vi "EncoderForward.vi"(8 "EncoderDevRef 4":T2={"DevStatus"={"status"=FALSE, "code"=0, "source"=""}, "EncoderIndex"=enum."Invalid", "CounterIndex"=enum."Ctr 1", "DistancePerCount"=2.0, "Decoding Type"=enum."4x"}, 9 "RobotDriveDevRef":T6={"DevStatus"={"status"=FALSE, "code"=0, "source"=""}, "Motors[]"=[], "Square Inputs"=FALSE, "Max Output"=1.0, "Isochronous"=FALSE}, 10 "EncoderDevRef":T2={"DevStatus"={"status"=FALSE, "code"=0, "source"=""}, "EncoderIndex"=enum."Invalid", "CounterIndex"=enum."Ctr 1", "DistancePerCount"=2.0, "Decoding Type"=enum."4x"}, 11 "Target":dbl format="%#_13g") -> (0 "EncoderDevRef 3":T2={"DevStatus"={"status"=FALSE, "code"=0, "source"=""}, "EncoderIndex"=enum."Invalid", "CounterIndex"=enum."Ctr 1", "DistancePerCount"=2.0, "Decoding Type"=enum."4x"}, 1 "RobotDriveDevRef 2":T6={"DevStatus"={"status"=FALSE, "code"=0, "source"=""}, "Motors[]"=[], "Square Inputs"=FALSE, "Max Output"=1.0, "Isochronous"=FALSE}, 2 "EncoderDevRef 2":T2={"DevStatus"={"status"=FALSE, "code"=0, "source"=""}, "EncoderIndex"=enum."Invalid", "CounterIndex"=enum."Ctr 1", "DistancePerCount"=2.0, "Decoding Type"=enum."4x"})   [LabVIEW 2013]
uses:
  <vilib>/Rock Robotics/WPI/RobotDrive/WPI_RobotDriveDevRef.ctl
  <vilib>/Rock Robotics/WPI/MotorControl/WPI_MotorControlDeviceRef.ctl
  <vilib>/Rock Robotics/SystemInterfaces/Typedef/FPGA_TypedefDigitalModule.ctl
  <vilib>/Rock Robotics/SystemInterfaces/DIO/FPGA_DIOPWMChannel.ctl
  <vilib>/Rock Robotics/WPI/PWM/WPI_PWMDeadband.ctl
  <vilib>/Rock Robotics/WPI/CAN/Jaguar/SubVIs/WPI_CANJaguar_ControlMode.ctl
  <vilib>/Rock Robotics/WPI/PWM/WPI_PWMTransform_ConPane.ctl
  <vilib>/Rock Robotics/WPI/Encoder/WPI_EncoderDevRef.ctl
  <vilib>/Rock Robotics/SystemInterfaces/Encoder/FPGA_EncoderIdx.ctl
  <vilib>/Rock Robotics/SystemInterfaces/Counter/FPGA_CounterCtrSystemIndex.ctl
  <vilib>/Rock Robotics/WPI/Encoder/WPI_EncoderType.ctl
  <vilib>/addons/control/pid/pid.llb/PID (DBL).vi
  <vilib>/addons/control/pid/NI_PID_pid.lvlib
panel:
  out "dt out (s)":dbl format="%.3f"
  out "Right Distance":dbl(graph)
  out "Right Motor Power":dbl(graph)
  out "Left Motor Power":dbl(graph)
  out "Left Distance":dbl(graph)
  in  "PID gains 3":T1={"proportional gain (Kc)"=0.15, "integral time (Ti, min)"=0.0, "derivative time (Td, min)"=0.0}
  in  "output range 3":cluster{"output high":dbl, "output low":dbl}={"output high"=1.0, "output low"=-1.0}
  in  "output range 2":cluster{"output high":dbl, "output low":dbl}={"output high"=1.0, "output low"=-1.0}
  in  "PID gains 2":T1={"proportional gain (Kc)"=0.15, "integral time (Ti, min)"=0.0, "derivative time (Td, min)"=0.0}
  # "Stop?"
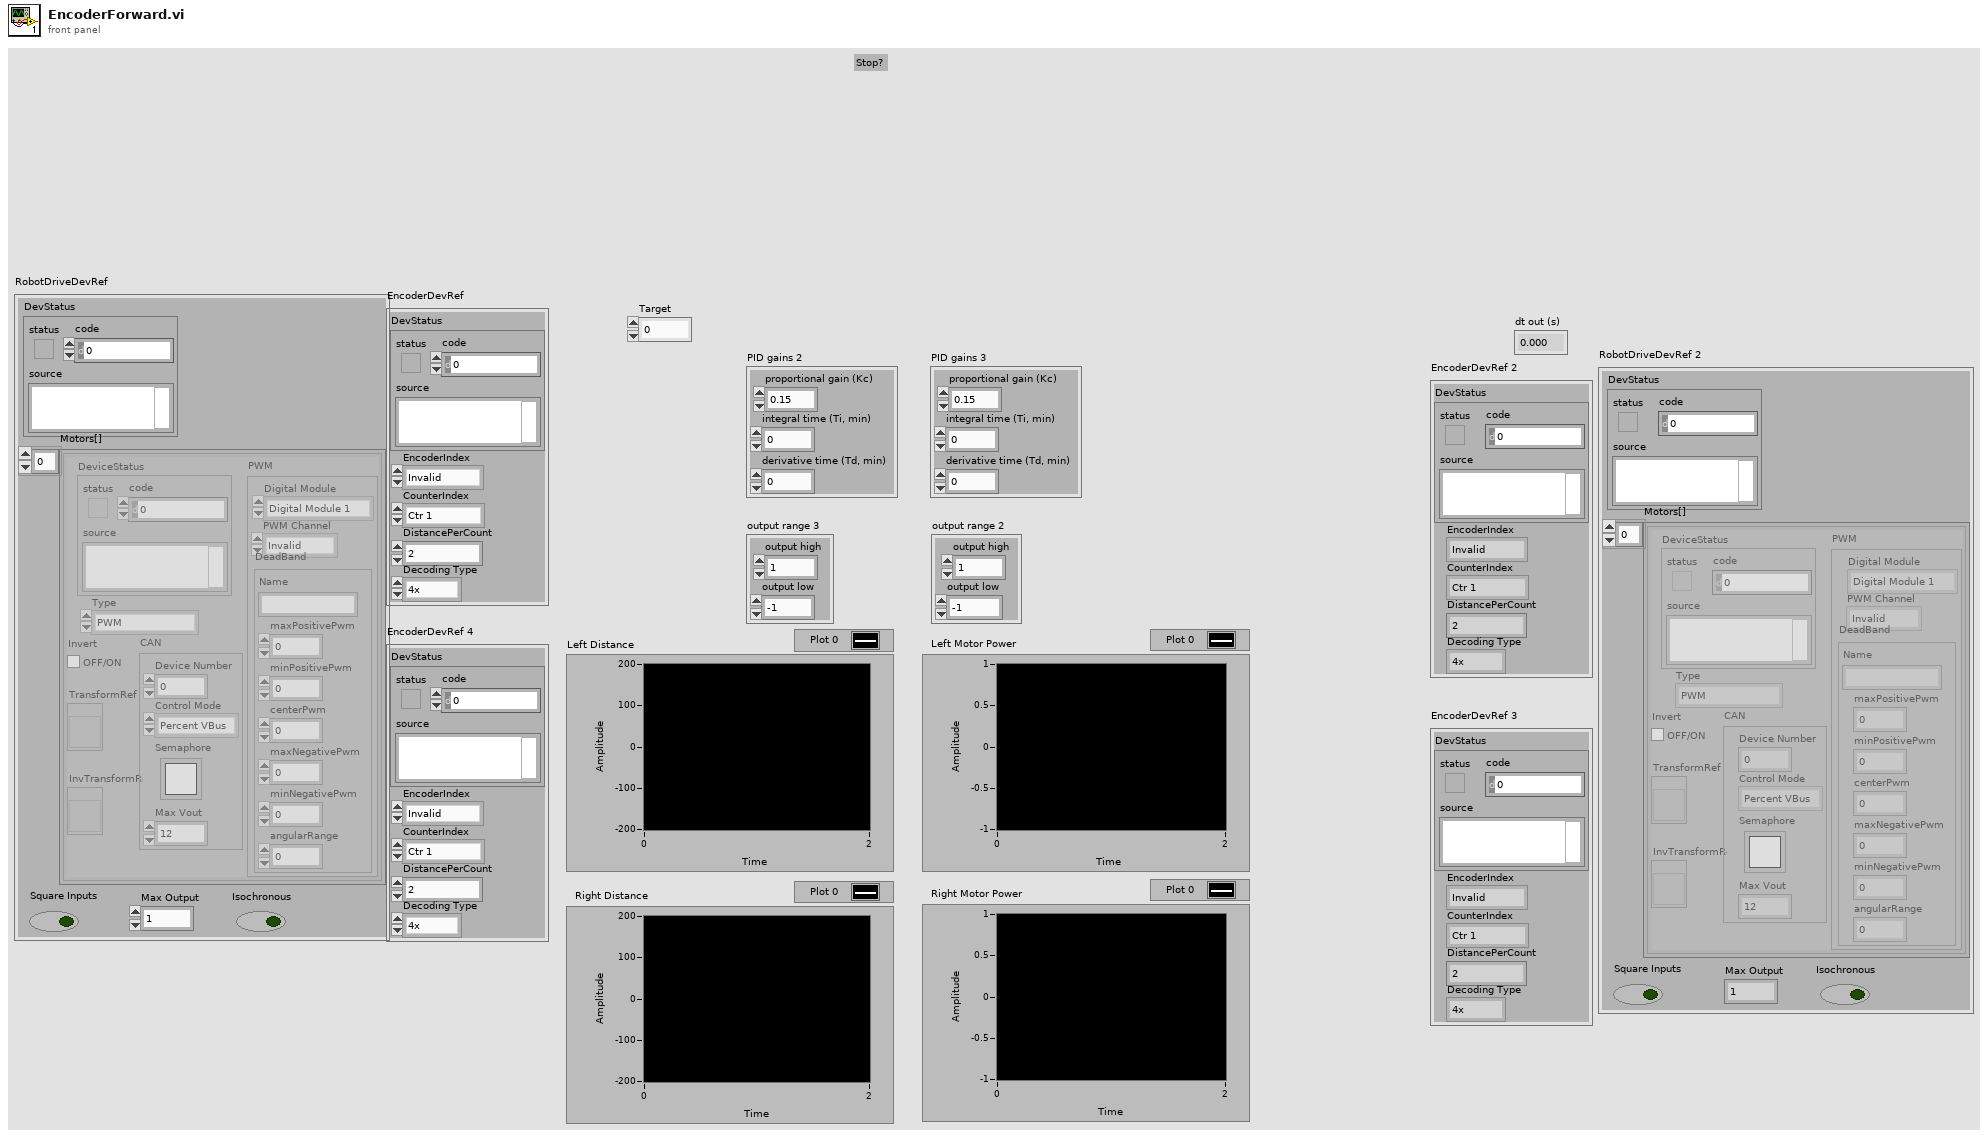
[diagram p1: front panel]
types:
  T1 = cluster{"proportional gain (Kc)":dbl, "integral time (Ti, min)":dbl, "derivative time (Td, min)":dbl}
  T2 = typedef "WPI_EncoderDevRef.ctl" = cluster{"DevStatus":errorcluster, "EncoderIndex":T3, "CounterIndex":T4, "DistancePerCount":dbl, "Decoding Type":T5}
  T3 = typedef "FPGA_EncoderIdx.ctl" = enum8{"Enc 0", "Enc 1", "Enc 2", "Enc 3", "Invalid"}
  T4 = typedef "FPGA_CounterCtrSystemIndex.ctl" = enum8{"Ctr 0", "Ctr 1", "Ctr 2", "Ctr 3", "Ctr 4", "Ctr 5", "Ctr 6", "Ctr 7", "Invalid"}
  T5 = typedef "WPI_EncoderType.ctl" = enum16{"1x", "2x", "4x"}
  T6 = typedef "WPI_RobotDriveDevRef.ctl" = cluster{"DevStatus":errorcluster, "Motors[]":T7[], "Square Inputs":bool, "Max Output":dbl, "Isochronous":bool}
  T7 = typedef "WPI_MotorControlDeviceRef.ctl" = cluster{"DeviceStatus":errorcluster, "Type":enum16{"PWM", "CAN"}, "PWM":cluster{"Digital Module":T8, "PWM Channel":T9, "DeadBand":T10}, "CAN":cluster{"Device Number":u8, "Control Mode":T11, "Semaphore":T12, "Max Vout":dbl}, "Invert":bool, "TransformRef":T13, "InvTransformRef":T13}
  T8 = typedef "FPGA_TypedefDigitalModule.ctl" = enum16{"Digital Module 1", "Digital Module 2"}
  T9 = typedef "FPGA_DIOPWMChannel.ctl" = enum8{"PWM 1", "PWM 2", "PWM 3", "PWM 4", "PWM 5", "PWM 6", "PWM 7", "PWM 8", "PWM 9", "PWM 10", "Invalid"}
  T10 = typedef "WPI_PWMDeadband.ctl" = cluster{"Name":string, "maxPositivePwm":i32, "minPositivePwm":i32, "centerPwm":i32, "maxNegativePwm":i32, "minNegativePwm":i32, "angularRange":u16}
  T11 = typedef "WPI_CANJaguar_ControlMode.ctl" = enum8{"Percent VBus", "Current", "Speed", "Position", "Voltage"}
  T12 = typedef "Semaphore RefNum" = refnum<k1>
  T13 = typedef "WPI_PWMTransform_ConPane.ctl" = refnum<vi>
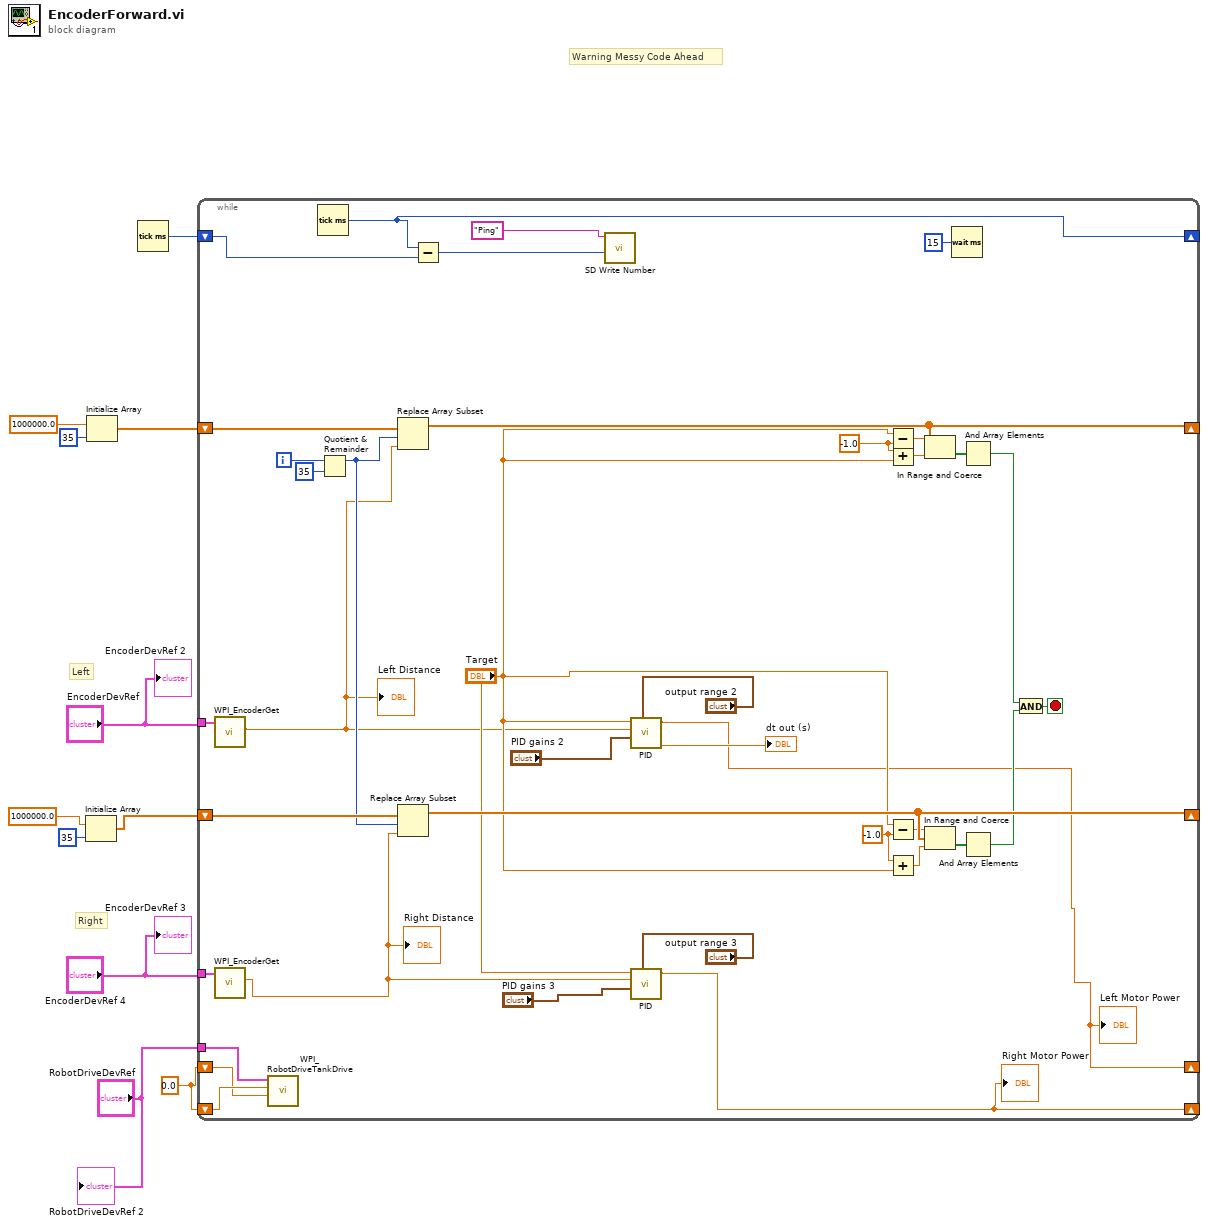
[diagram p0: block diagram]
diagram:
  w3 = 0.0 ("output")
  # "Warning Messy Code Ahead"
  # "Right"
  # "Left"
  n1 = Initialize Array(1000000.0 ("element"), 35 ("dimension size")) -> (w6:dbl[])
  n2 = Initialize Array(1000000.0 ("element"), 35 ("dimension size")) -> (w7:dbl[])
  n3 = Tick Count (ms)() -> (millisecond timer value=w11:u32)
  n4 = while {
    shift-right: [w47] -> _
    shift-left: w11 -> [w48]
    shift-right: [w15] -> _
    shift-left: w3 -> [w21]
    tunnel: "RobotDriveDevRef" -> [w46]
    shift-right: [w20] -> _
    shift-left: w7 -> [w43]
    tunnel: "EncoderDevRef" -> [w35]
    shift-right: [w31] -> _
    shift-left: w6 -> [w28]
    tunnel: "EncoderDevRef 4" -> [w34]
    shift-right: [w14] -> _
    shift-left: w3 -> [w22]
    i -> [w39]
    stop <- w26 stop-if-true
    w33 = -1.0 ("y")
    w36 = -1.0 ("y")
    n5 = call <vilib>:"WPI_EncoderGet.vi"("EncoderDevRef"=w35) -> ("Distance"=w16:dbl)  [unwired: 1 in, 9 out]
    "Left Distance" <- w16
    n6 = call <vilib>:"WPI_EncoderGet.vi"("EncoderDevRef"=w34) -> ("Distance"=w17:dbl)  [unwired: 1 in, 9 out]
    "Right Distance" <- w17
    n7 = call <vilib>:"WPI_RobotDriveTankDrive.vi"("Right axis value"=w21, "Left axis value"=w22, "RobotDriveDevRef"=w46) -> ()  [unwired: 6 in, 3 out]
    n8 = Tick Count (ms)() -> (millisecond timer value=w47:u32)
    n9 = Quotient & Remainder(x=w39, y=35) -> (x-y*floor(x/y)=w23:i32)  [unwired: 1 out]
    n10 = Replace Array Subset(array=w43, new element=w16, index=w23) -> (w20:dbl[])
    n11 = Replace Array Subset(array=w28, new element=w17, index=w23) -> (w31:dbl[])
    n12 = Subtract(x=w47, y=w48) -> (x-y=w40:u32)
    n13 = call <vilib>:"SD Write Number.vi"("Numeric"=w40, "Name"="Ping") -> ()  [unwired: 8 in, 2 out]
    n14 = call-poly <vilib>:"PID.vi"("output range"="output range 2", "PID gains"="PID gains 2", "process variable"=w16, "setpoint"="Target") -> ("dt out (s)"=→"dt out (s)":dbl, "output"=w15:dbl)  [unwired: 6 in]
    "Left Motor Power" <- w15
    n15 = call-poly <vilib>:"PID.vi"("output range"="output range 3", "PID gains"="PID gains 3", "process variable"=w17, "setpoint"="Target") -> ("output"=w14:dbl)  [unwired: 6 in, 1 out]
    "Right Motor Power" <- w14
    n16 = Subtract(x="Target", y=w36) -> (x-y=w42:dbl)
    n17 = Add(x=w36, y="Target") -> (x+y=w37:dbl)
    n18 = Subtract(x="Target", y=w33) -> (x-y=w29:dbl)
    n19 = Add(x=w33, y="Target") -> (x+y=w32:dbl)
    n20 = In Range and Coerce(upper limit=w42, x=w20, lower limit=w37) -> (In Range?=w38:bool[])  [unwired: 1 out]
    n21 = In Range and Coerce(upper limit=w29, x=w31, lower limit=w32) -> (In Range?=w30:bool[])  [unwired: 1 out]
    n22 = Wait (ms)(milliseconds to wait=u32 15) -> ()  [unwired: 1 out]
    n23 = And Array Elements(Boolean array=w38) -> (logical AND=w25:bool)
    n24 = And Array Elements(Boolean array=w30) -> (logical AND=w24:bool)
    n25 = And(x=w25, y=w24) -> (x .and. y?=w26:bool)
  }
  "RobotDriveDevRef 2" <- "RobotDriveDevRef"
  "EncoderDevRef 2" <- "EncoderDevRef"
  "EncoderDevRef 3" <- "EncoderDevRef 4"
